vi "TS Acq Start.vi"(8 "error in":errorcluster, 11 "Test Stand in":refnum<class "Cryo Sep Test Stand.lvclass">) -> (0 "error out":errorcluster, 3 "Test Stand out":refnum<class "Cryo Sep Test Stand.lvclass">)   [LabVIEW 2019, in "Test Stands.lvlib" / "Cryo Sep Test Stand.lvclass"]
uses:
  Cryo Sep Test Stand.lvclass
  <vilib>/DAQmx/write.llb/DAQmx Write (Analog DBL 1Chan 1Samp).vi
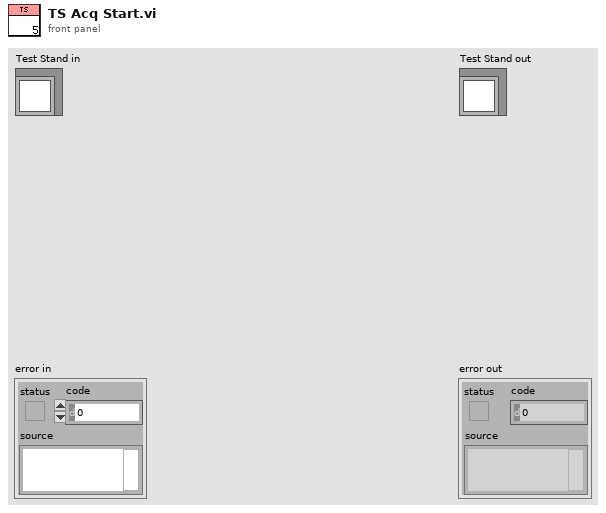
[diagram p1: front panel]
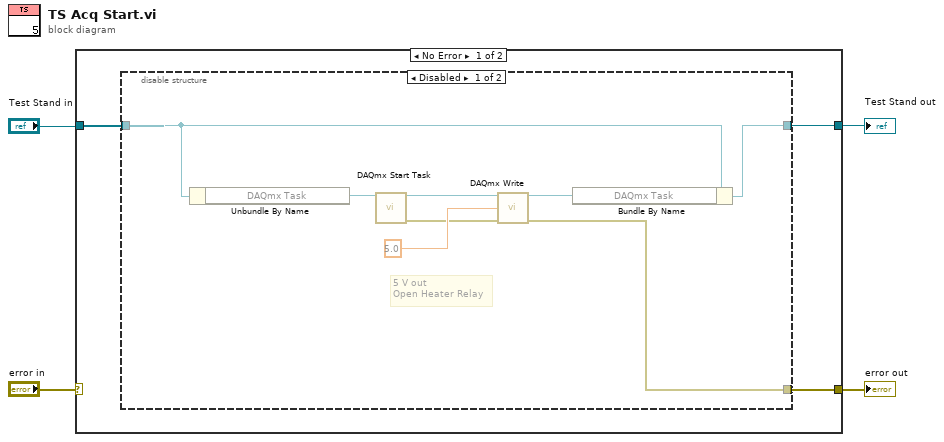
[diagram p0: block diagram]
diagram:
  n1 = case shown="No Error" "error in" {
    selector: "error in" -> [_ w18]
    tunnel: [w5 w18] -> w1
    tunnel: [w6 w17] -> w3
    tunnel: "Test Stand in" -> [w7 w17]
    frame No Error {
      n2 = disable-structure shown="Disabled" {
        disable-tunnel: w7 -> [w11 w16]
        disable-tunnel: [w9 w16] -> w6
        disable-tunnel: [w8 _] -> w5
        frame Disabled {
          # "5 V out\nOpen Heater Relay"
          n3 = Unbundle By Name(w11) -> ("DAQmx Task"=w15:refnum<k21>)
          n4 = call <vilib>:"DAQmx Start Task.vi"("task/channels in"=w15) -> ("task out"=w14:refnum<k21>, "error out"=w12:errorcluster)  [unwired: 13 in]
          n5 = call-poly <vilib>:"DAQmx Write.vi"("task/channels in"=w14, "data"=5.0, "error in"=w12) -> ("task out"=w10:refnum<k21>, "error out"=w8:errorcluster)  [unwired: 10 in, 1 out]
          n6 = Bundle By Name(cluster=w11, "DAQmx Task"=w10) -> (w9:refnum<class "Cryo Sep Test Stand.lvclass">)
        }
        frame Enabled {
        }
      }
    }
    frame Error {
    }
  }
  "error out" <- w1
  "Test Stand out" <- w3
